vi "OFDM_RFLoopback.vi"(0 "PathIn":path, 1 "rfflag":dbl, 2 "EN_Mutipath":dbl, 3 "EN_NOISE":dbl, 4 "EN_TIMEOFFSET":dbl, 5 "lenburstinter":dbl, 7 "SNR":dbl, 8 "timeoffset":dbl, 9 "EN_BUTSRINTER":dbl, 10 "mutitimeoffset":dbl[](array[numeric]), 11 "mutifreoffset":dbl[](array[numeric]), 12 "recant":dbl, 13 "EN_FREOFFSET":dbl, 14 "txantnum":dbl, 15 "atte_factor":dbl, 16 "txindex":dbl, 17 "error in (no error)":errorcluster caption="错误输入（无错误）", 18 "mutiamp":dbl[](array[numeric]), 19 "mutiphaseoffset":dbl[](array[numeric]), 20 "txdata":cdb[](array[numeric]), 21 "freoffset":dbl, 23 "pcip":string, 24 "xsrpip":string) -> (25 "rxdata":cdb[](array[numeric]), 27 "error out":errorcluster caption="错误输出")   [LabVIEW 2015]
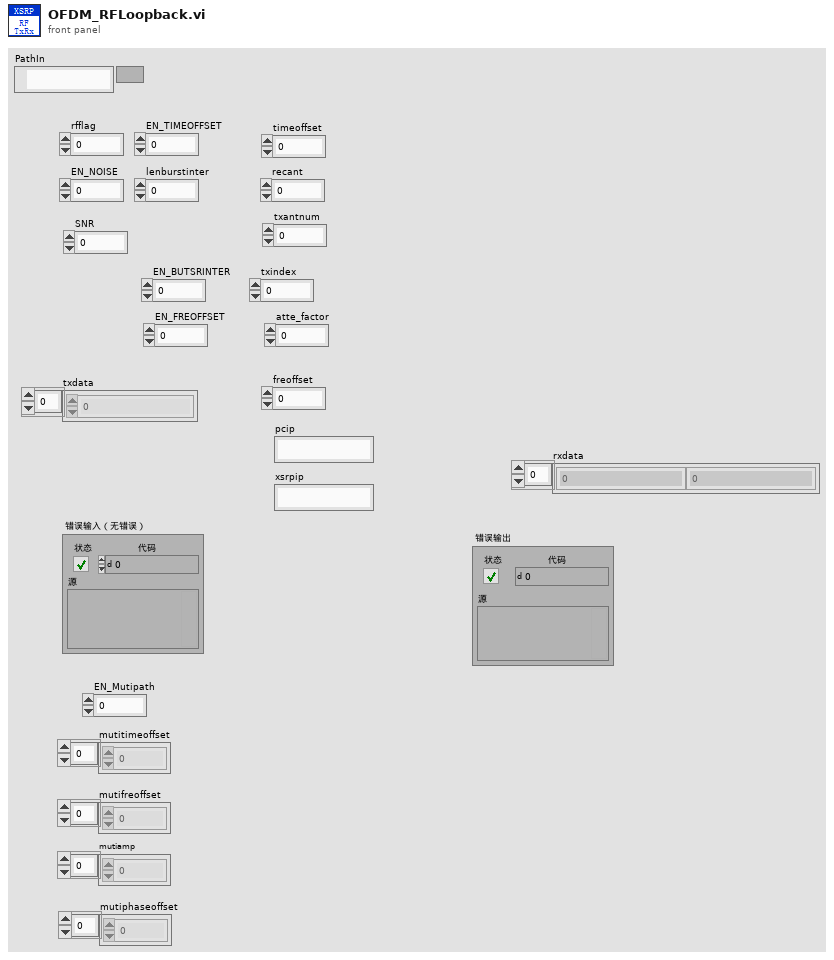
[diagram p1: front panel]
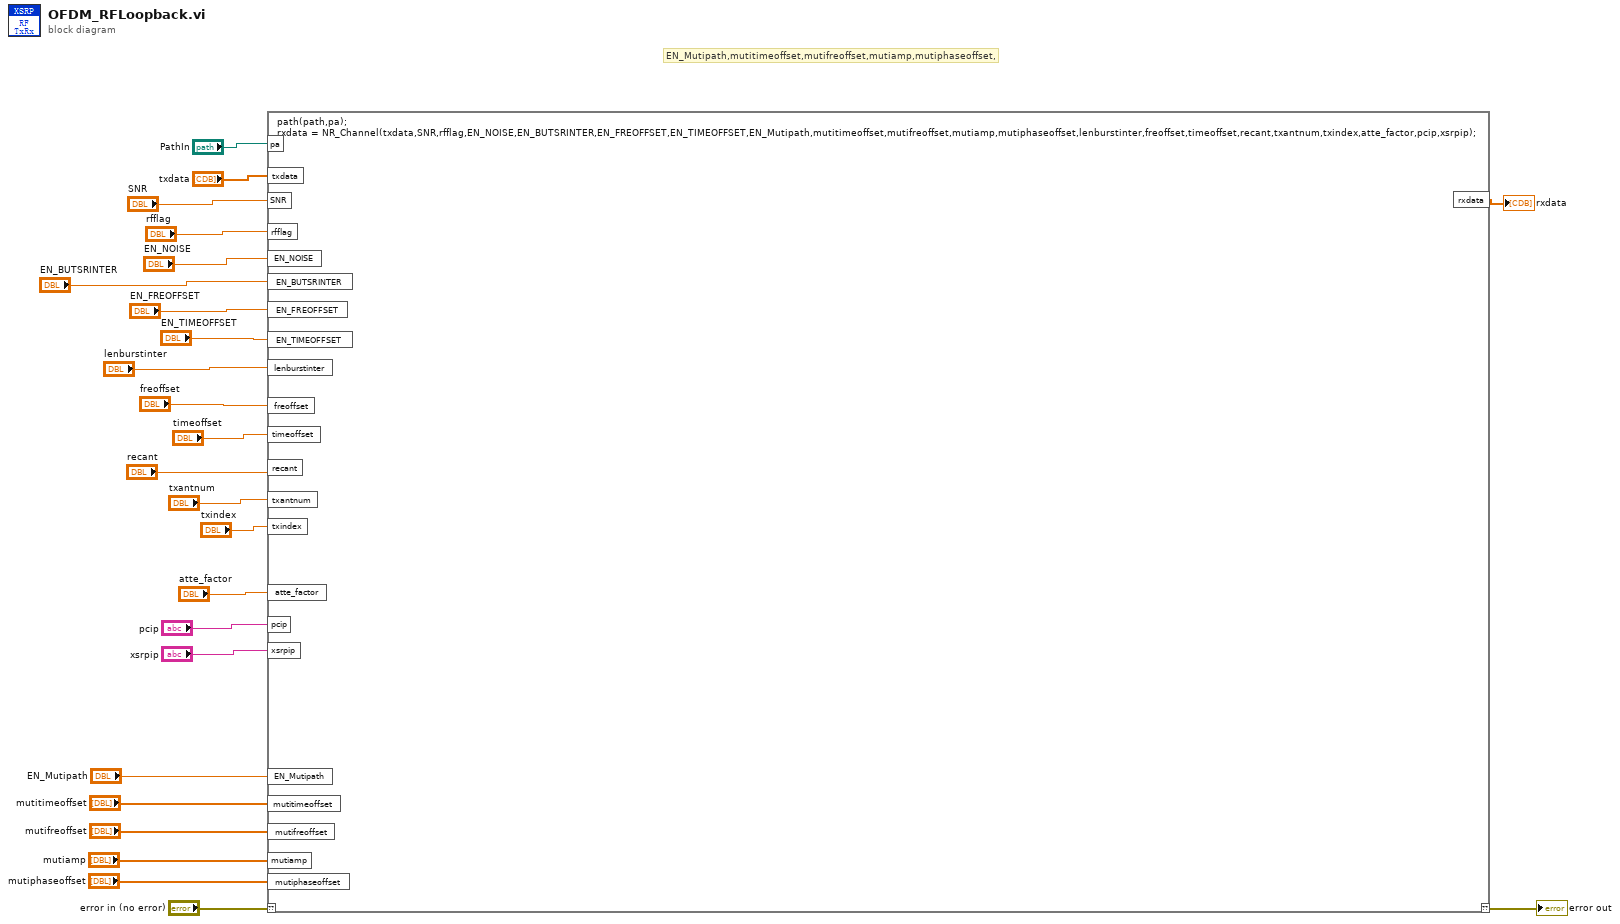
[diagram p0: block diagram]
diagram:
  # "EN_Mutipath,mutitimeoffset,mutifreoffset,mutiamp,mutiphaseoffset,"
  n1 = script code="path(path,pa);\nrxdata = NR_Channel(txdata,SNR,rfflag,EN_NOISE,EN_BUTSRINTER,EN_FREOFFSET,EN_TIMEOFFSET,EN_Mutipath,mutitimeoffset,mutifreoffset,mutiamp,mutiphaseoffset,lenburstinter,freoffset,timeoffset,recant,txantnum,txindex,atte_factor,pcip,xsrpip);"("??"="error in (no error)", "pa"="PathIn", "txdata"="txdata", "pcip"="pcip", "xsrpip"="xsrpip", "SNR"="SNR", "rfflag"="rfflag", "EN_NOISE"="EN_NOISE", "EN_BUTSRINTER"="EN_BUTSRINTER", "EN_FREOFFSET"="EN_FREOFFSET", "EN_TIMEOFFSET"="EN_TIMEOFFSET", "lenburstinter"="lenburstinter", "freoffset"="freoffset", "timeoffset"="timeoffset", "recant"="recant", "txantnum"="txantnum", "txindex"="txindex", "atte_factor"="atte_factor", "EN_Mutipath"="EN_Mutipath", "mutitimeoffset"="mutitimeoffset", "mutifreoffset"="mutifreoffset", "mutiamp"="mutiamp", "mutiphaseoffset"="mutiphaseoffset") -> ("??"=→"error out":errorcluster, "rxdata"=→"rxdata":cdb[])
